vi "Labview Plots.vi"(9 "3d Graph Selector":u16(ring) items=["Error Plot", "Measured Data", "Path Plot", "Reference"]) -> (1 "surface":refnum<class "3D Plot Datatype.lvclass">[](array[class]), 2 "comet":refnum<class "3D Plot Datatype.lvclass">[](array[class]))   [LabVIEW 2017]
uses:
  <vilib>/Math Plots/3D Math Plots/3D Plot/3D Plot Datatype/3D Plot Datatype.lvclass
  <vilib>/Math Plots/3D Math Plots/3D Surface/3D Surface XCtrl/3D Surface.xctl
  Globals.vi
  <vilib>/Math Plots/3D Math Plots/3D Surface/3D Surface Datatype/Public/Plot Helper (Matrix).vi
  <vilib>/Math Plots/3D Math Plots/3D Comet/3D Comet Datatype/Public/Plot Helper (Vector).vi
  <vilib>/Math Plots/3D Math Plots/3D Surface/3D Surface Datatype/3D Surface Datatype.lvclass
  <vilib>/Math Plots/3D Math Plots/3D Comet/3D Comet Datatype/3D Comet Datatype.lvclass
panel:
  out "error out 8":errorcluster
  out "error out 7":errorcluster
  out "error out 6":errorcluster
  out "error out 5":errorcluster
  out "error out 4":errorcluster
  out "error out 3":errorcluster
  out "error out 2":errorcluster
  out "error out":errorcluster
  out "3D Surface":refnum<class "3D Plot Datatype.lvclass">[](xcontrol)
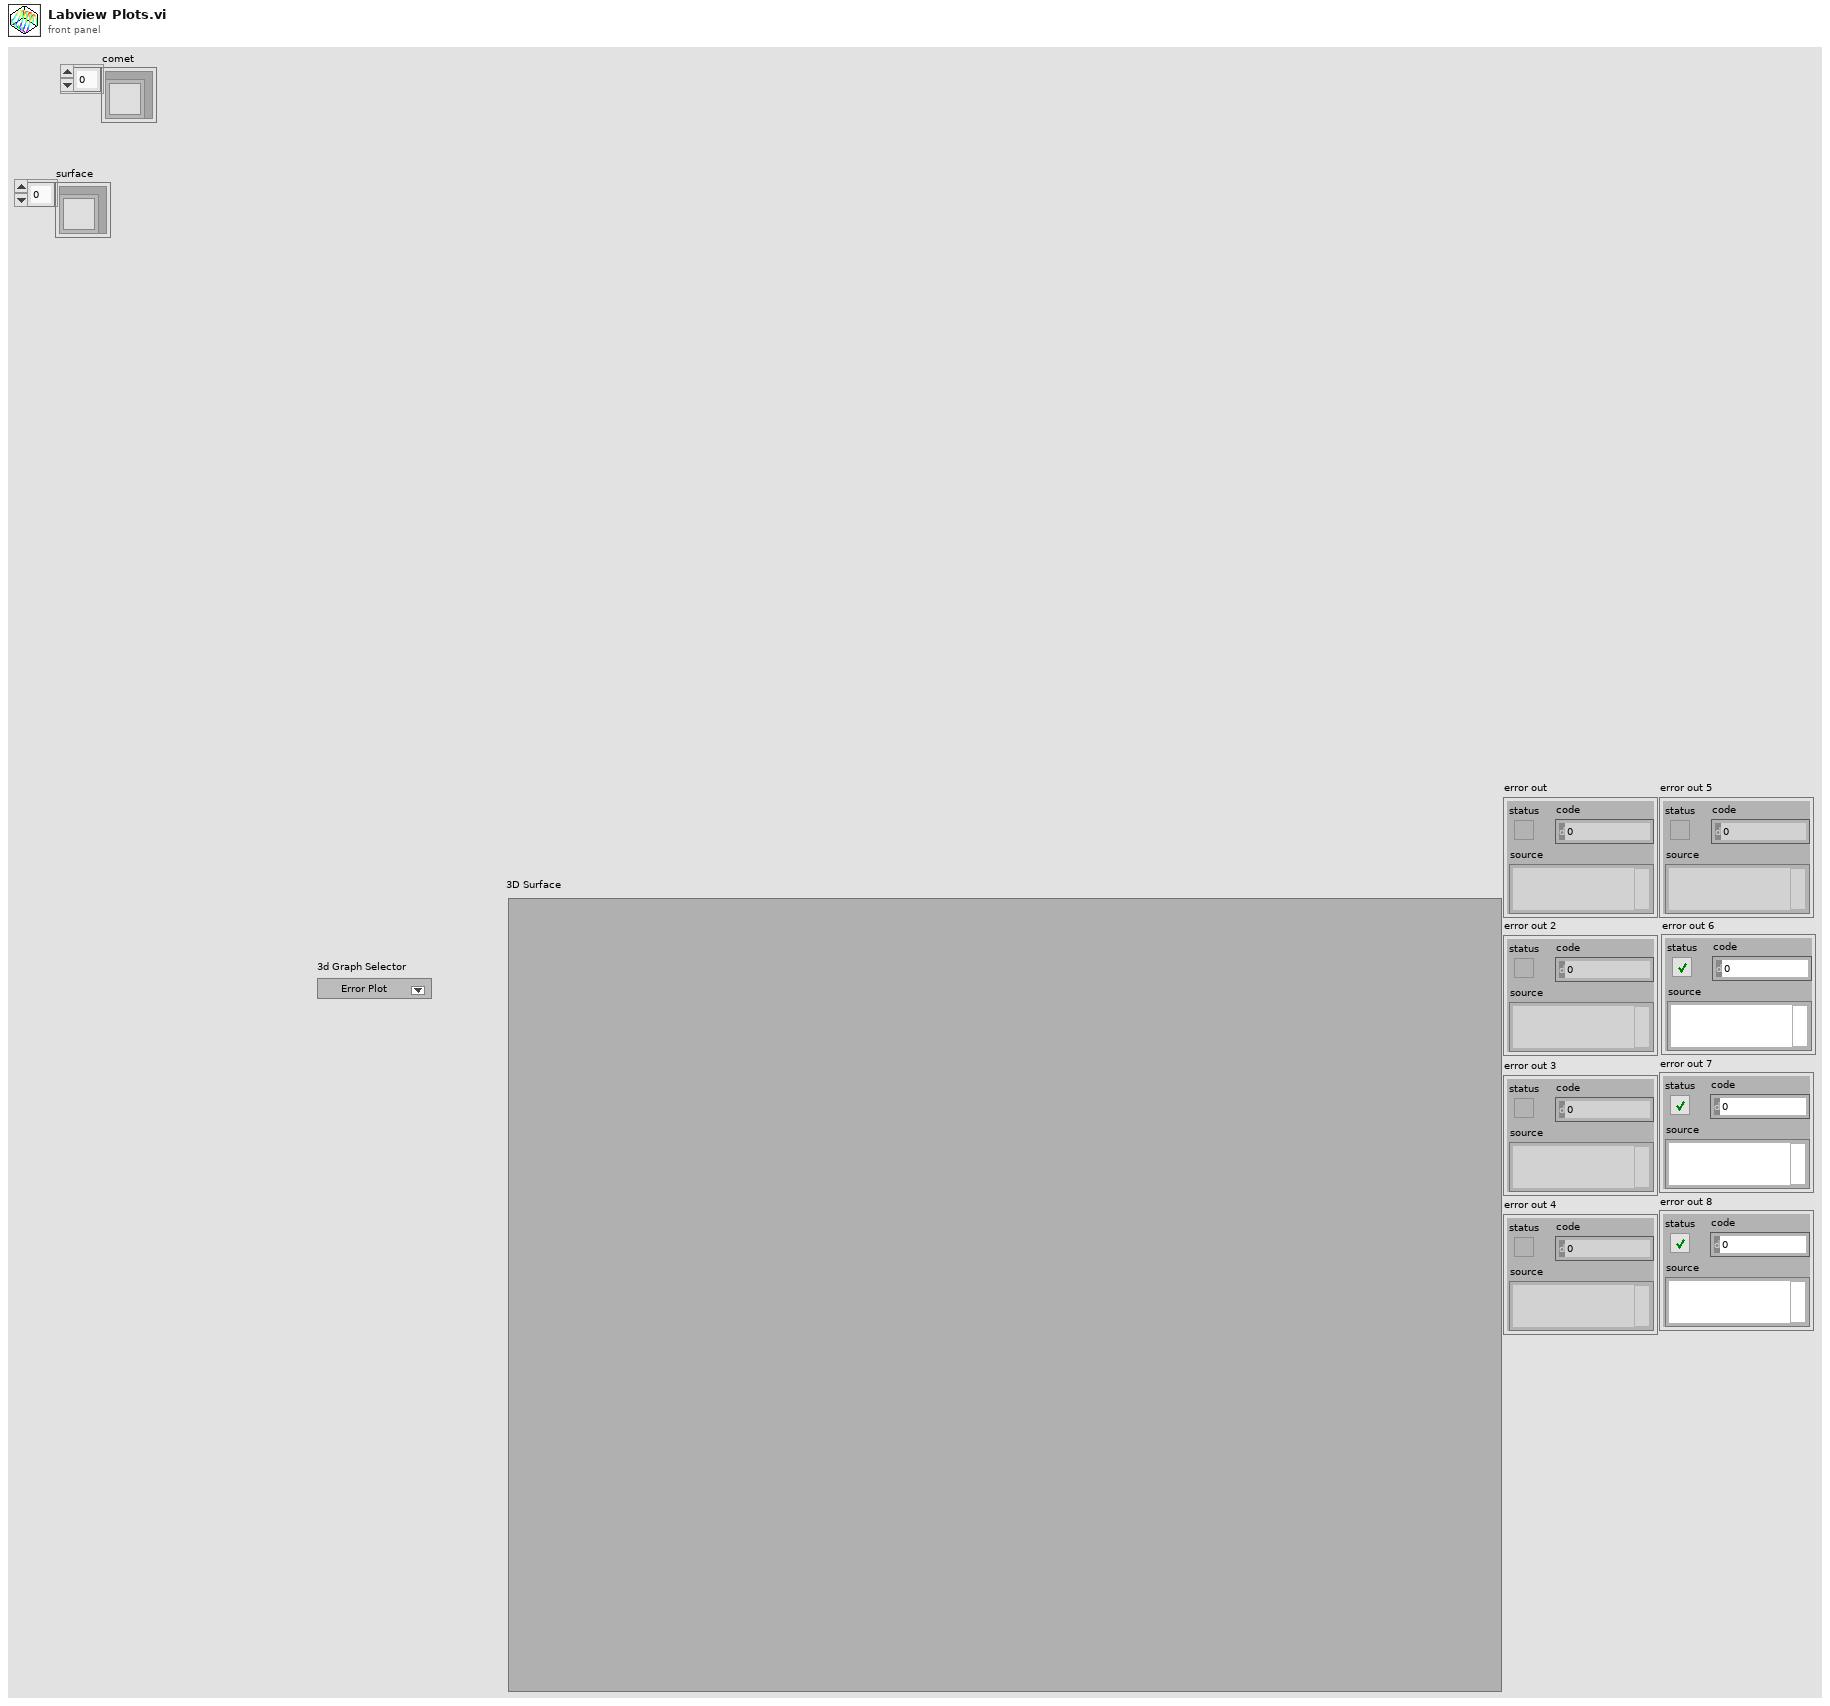
[diagram p1: front panel]
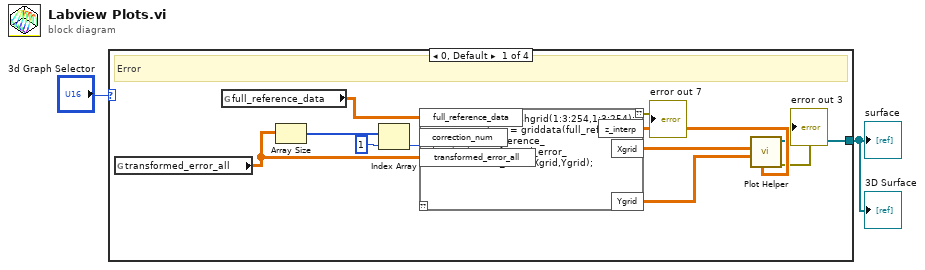
[diagram p0: block diagram]
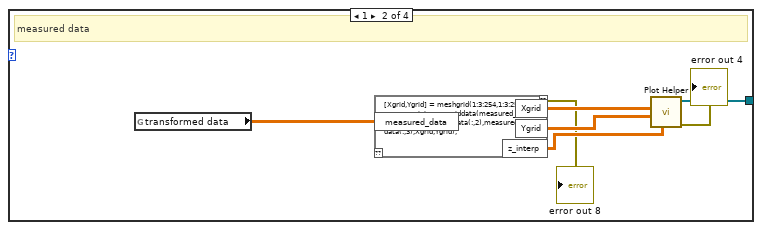
[diagram p2: hidden frame]
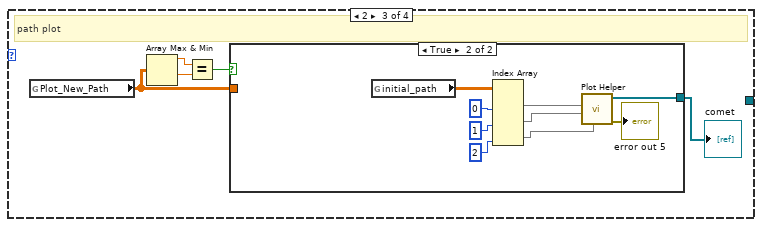
[diagram p3: hidden frame]
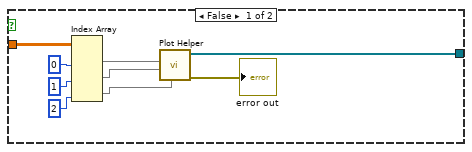
[diagram p4: hidden frame]
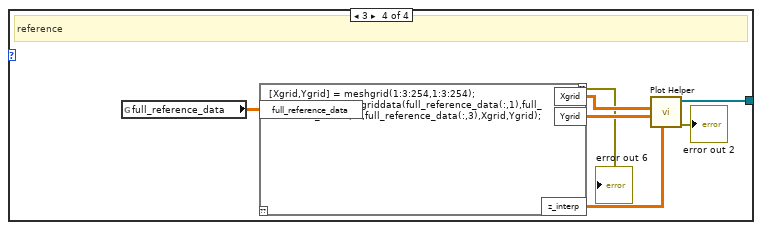
[diagram p5: hidden frame]
diagram:
  n1 = case shown="0, Default" "3d Graph Selector" {
    tunnel: [w9 w19 _ w46] -> w1
    frame 0, Default {
      # "Error"
      n2 = global read "Globals.vi" "transformed_error_all"() -> (w8:dbl[][])
      n3 = global read "Globals.vi" "full_reference_data"() -> (w10:dbl[][])
      n4 = Array Size(array=w8) -> (size(s)=w7:i32[])
      n5 = Index Array(array=w7, index=1) -> (element=w5:i32)
      n6 = script code="[Xgrid,Ygrid] = meshgrid(1:3:254,1:3:254);\n             z_interp = griddata(full_reference_data(:,1),full_reference_data(:,2),transformed_error_all(:,correction_num),Xgrid,Ygrid);" ("Script Node")("full_reference_data"=w10, "transformed_error_all"=w8, "correction_num"=w5) -> ("??"=→"error out 7":errorcluster, "Xgrid"=w13:dbl[][], "Ygrid"=w12:dbl[][], "z_interp"=w11:dbl[][])  [unwired: 1 in]
      n7 = call-poly <vilib>:"Plot Helper.vi"("z matrix"=w11, "y matrix"=w12, "x matrix"=w13) -> ("error out"=→"error out 3":errorcluster, "3D Plot lvclass Array out"=w9:refnum<class "3D Plot Datatype.lvclass">[])  [unwired: 3 in, 4 out]
    }
    frame 1 {
      # "measured data"
      n8 = global read "Globals.vi" "transformed data"() -> (w20:dbl[][])
      n9 = script code="[Xgrid,Ygrid] = meshgrid(1:3:254,1:3:254);\n             z_interp = griddata(measured_data(:,1),measured_data(:,2),measured_data(:,3),Xgrid,Ygrid);" ("Script Node")("measured_data"=w20) -> ("??"=→"error out 8":errorcluster, "Xgrid"=w18:dbl[][], "Ygrid"=w17:dbl[][], "z_interp"=w16:dbl[][])  [unwired: 1 in]
      n10 = call-poly <vilib>:"Plot Helper.vi"("z matrix"=w16, "y matrix"=w17, "x matrix"=w18) -> ("error out"=→"error out 4":errorcluster, "3D Plot lvclass Array out"=w19:refnum<class "3D Plot Datatype.lvclass">[])  [unwired: 3 in, 4 out]
    }
    frame 2 {
      # "path plot"
      n11 = global read "Globals.vi" "Plot_New_Path"() -> (w22:dbl[][])
      n12 = Array Max & Min(array=w22) -> (max value=w24:dbl, min value=w25:dbl)  [unwired: 2 out]
      n13 = Equal?(x=w24, y=w25) -> (x = y?=w23:bool)
      n14 = case shown="True" w23 {
        tunnel: w22 -> [w28 _]
        tunnel: [w27 w37] -> w21
        frame False {
          n15 = Index Array(array=w28, index (col) #1=0 ("disabled index (col)"), index (col) #2=1 ("disabled index (col)"), index (col) #3=2 ("index (col)")) -> (element #1=w31:dbl[], element #2=w30:dbl[], element #3=w29:dbl[])  [unwired: 3 in]
          n16 = call-poly <vilib>:"Plot Helper.vi"("z vector"=w29, "y vector"=w30, "x vector"=w31) -> ("error out"=→"error out":errorcluster, "3D Plot lvclass Array out"=w27:refnum<class "3D Plot Datatype.lvclass">[])  [unwired: 3 in, 4 out]
        }
        frame True {
          n17 = global read "Globals.vi" "initial_path"() -> (w36:dbl[][])
          n18 = Index Array(array=w36, index (col) #1=0 ("disabled index (col)"), index (col) #2=1 ("disabled index (col)"), index (col) #3=2 ("index (col)")) -> (element #1=w40:dbl[], element #2=w39:dbl[], element #3=w38:dbl[])  [unwired: 3 in]
          n19 = call-poly <vilib>:"Plot Helper.vi"("z vector"=w38, "y vector"=w39, "x vector"=w40) -> ("error out"=→"error out 5":errorcluster, "3D Plot lvclass Array out"=w37:refnum<class "3D Plot Datatype.lvclass">[])  [unwired: 3 in, 4 out]
        }
      }
      "comet" <- w21
    }
    frame 3 {
      # "reference"
      n20 = global read "Globals.vi" "full_reference_data"() -> (w50:dbl[][])
      n21 = script code="[Xgrid,Ygrid] = meshgrid(1:3:254,1:3:254);\n             z_interp = griddata(full_reference_data(:,1),full_reference_data(:,2),full_reference_data(:,3),Xgrid,Ygrid);" ("Script Node")("full_reference_data"=w50) -> ("??"=→"error out 6":errorcluster, "Xgrid"=w49:dbl[][], "Ygrid"=w48:dbl[][], "z_interp"=w47:dbl[][])  [unwired: 1 in]
      n22 = call-poly <vilib>:"Plot Helper.vi"("z matrix"=w47, "y matrix"=w48, "x matrix"=w49) -> ("error out"=→"error out 2":errorcluster, "3D Plot lvclass Array out"=w46:refnum<class "3D Plot Datatype.lvclass">[])  [unwired: 3 in, 4 out]
    }
  }
  "surface" <- w1
  "3D Surface" <- w1
